vi "Read-Write To-From Text File.vi"(6 "string to be written":string, 7 "dialog box prompt":string, 8 "error in (no error)":errorcluster, 9 "file name (read description)":path, 10 "read/write (f:read)":bool, 11 "default path (read description)":path) -> (0 "error out":errorcluster, 1 "string which was read":string)   [LabVIEW 2018, in "Agilent 87XX Series.lvlib"]
doc: "This VI was designed to be used with the HP8753B Network Analyzer for reading and writing strings to and from the disk. There\nis not to much in here that can not be found in the other file VIs. This VI allows a default file path and dialog box to be set. It also allows the user to enter a special dialog box prompt.\n\n If a file is selected to be written to which already exists, the user will be queried if s/he really wants to overwrite the file.\n\n Refer to the LabVIEW Function Reference Manual for complete details on text files."
uses:
  Agilent 87XX Series.lvlib
panel:
  # "write to file\nread from file"
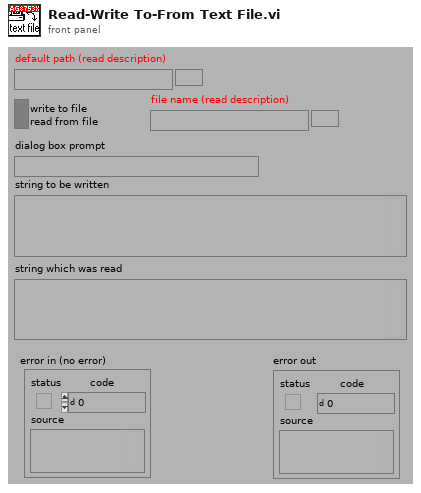
[diagram p1: front panel]
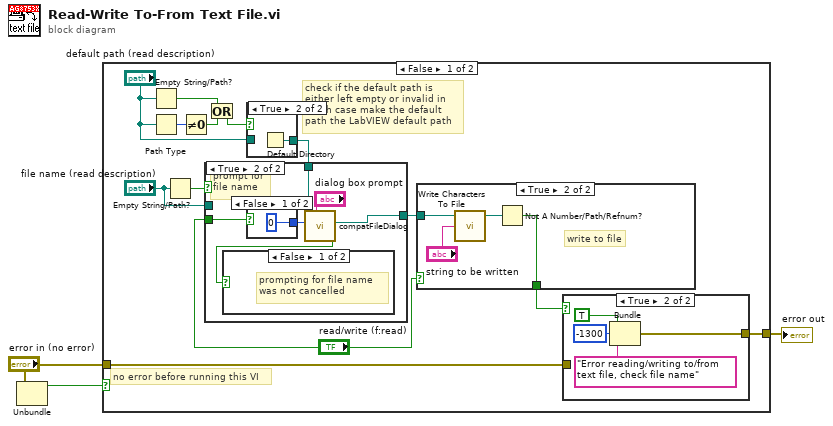
[diagram p0: block diagram]
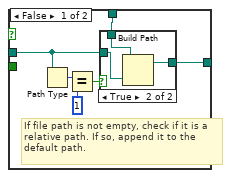
[diagram p3: hidden frame]
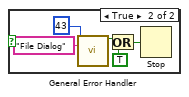
[diagram p5: hidden frame]
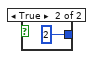
[diagram p6: hidden frame]
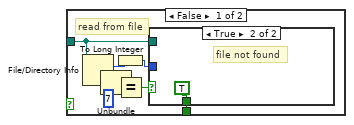
[diagram p7: hidden frame]
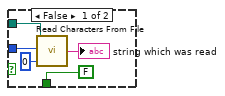
[diagram p8: hidden frame]
diagram:
  n1 = Unbundle("error in (no error)") -> ("status"=w2:bool)  [unwired: 2 out]
  n2 = case shown="False" w2 {
    tunnel: "error in (no error)" -> [w11 w65]
    tunnel: [w10 w65] -> w1
    frame False {
      # "check if the default path is either left empty or invalid in which case make the default path the LabVIEW default path"
      # "no error before running this VI"
      n3 = Empty String/Path?(string/path="default path (read description)") -> (empty?=w7:bool)
      n4 = Path Type(1:"default path (read description)") -> (0:w8:i16)
      n5 = Empty String/Path?(string/path="file name (read description)") -> (empty?=w14:bool)
      n6 = Not Equal To 0?(x=w8) -> (x != 0?=w6:bool)
      n7 = Or(x=w7, y=w6) -> (x .or. y?=w5:bool)
      n8 = case shown="True" w5 {
        tunnel: [w63 w64] -> w13
        tunnel: "default path (read description)" -> [w63 _]
        frame False {
        }
        frame True {
          n9 = Default Directory() -> (w64:path)
        }
      }
      n10 = case shown="True" w14 {
        tunnel: "read/write (f:read)" -> [_ w37]
        tunnel: w13 -> [w22 w35]
        tunnel: [w24 w34] -> w16
        tunnel: "file name (read description)" -> [w23 _]
        frame False {
          # "If file path is not empty, check if it is a\nrelative path. If so, append it to the \ndefault path."
          n11 = Path Type(1:w23) -> (0:w27:i16)
          n12 = Equal?(x=w27, y=i16 1) -> (x = y?=w25:bool)
          n13 = case shown="True" w25 {
            tunnel: [w28 w29] -> w24
            tunnel: w23 -> [w28 w30]
            tunnel: w22 -> [_ w31]
            frame False {
            }
            frame True {
              n14 = Build Path(base path=w31, name or relative path=w30) -> (appended path=w29:path)
            }
          }
        }
        frame True {
          # "prompt for\nfile name"
          n15 = case shown="False" w37 {
            tunnel: [i16 0 i16 2] -> w36
            frame False {
            }
            frame True {
            }
          }
          n16 = call <vilib>:"compatFileDialog.vi"("prompt"="dialog box prompt", "select mode (2)"=w36, "start path"=w35) -> ("cancelled"=w32:bool, "path"=w34:path)  [unwired: 6 in, 1 out]
          n17 = case shown="False" w32 {
            frame False {
              # "prompting for file name \nwas not cancelled"
            }
            frame True {
              n18 = call <vilib>:"General Error Handler.vi"("[error code] (0)"=43, "[error source] (\" \")"="File Dialog") -> ("error?"=w40:bool)  [unwired: 9 in, 4 out]
              n19 = Or(x=w40, y=TRUE) -> (x .or. y?=w38:bool)
              n20 = Stop(stop? (T)=w38) -> ()
            }
          }
        }
      }
      n21 = case shown="True" "read/write (f:read)" {
        tunnel: w16 -> [w48 w62]
        tunnel: [w49 w60] -> w4
        frame False {
          # "read from file"
          n22 = File/Directory Info(path=w48) -> (size=w45:i64, error out=w51:errorcluster)  [unwired: 1 in, 5 out]
          n23 = Unbundle(w51) -> ("code"=w46:i32)  [unwired: 2 out]
          n24 = To Long Integer(number=w45) -> (32bit integer=w47:i32)
          n25 = Equal?(x=w46, y=7) -> (x = y?=w50:bool)
          n26 = case shown="True" w50 {
            tunnel: [FALSE TRUE] -> w49
            tunnel: w48 -> [w54 _]
            tunnel: w47 -> [w53 _]
            frame False {
              n27 = call <vilib>:"Read Characters From File.vi"("file path (dialog if empty)"=w54, "number of characters (all:-1)"=w53, "start of read offset (chars.:0)"=0) -> ("character string"=→"string which was read":string)  [unwired: 3 in, 3 out]
            }
            frame True {
              # "file not found"
            }
          }
        }
        frame True {
          # "write to file"
          n28 = call <vilib>:"Write Characters To File.vi"("character string"="string to be written", "file path (dialog if empty)"=w62) -> ("new file path (Not A Path if cancelled)"=w59:path)  [unwired: 3 in]
          n29 = Not A Number/Path/Refnum?(number/path/refnum=w59) -> (NaN/Path/Refnum?=w60:bool)
        }
      }
      n30 = case shown="True" w4 {
        tunnel: [w17 w18] -> w10
        tunnel: w11 -> [w17 _]
        frame False {
          # "no error reading/writing"
        }
        frame True {
          n31 = Bundle(TRUE, -1300, "Error reading/writing to/from text file, check file name") -> (w18:errorcluster)  [unwired: 1 in]
        }
      }
    }
    frame True {
      # "an error has occurred before running this VI"
    }
  }
  "error out" <- w1
